vi "SetClipboardData.vi"(4 "error in (no error)":errorcluster, 6 "Format (CF_TEXT)":T1, 7 "hMem":i32 format="%.0x") -> (0 "error out":errorcluster, 3 "hData":i32 format="%.0x")   [LabVIEW 2011]
uses:
  Clipboard Formats.ctl
  KERNEL32.DLL
  user32.dll
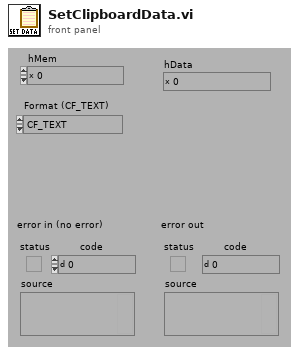
[diagram p1: front panel]
types:
  T1 = typedef "Clipboard Formats.ctl" = enum16{"CF_TEXT"}
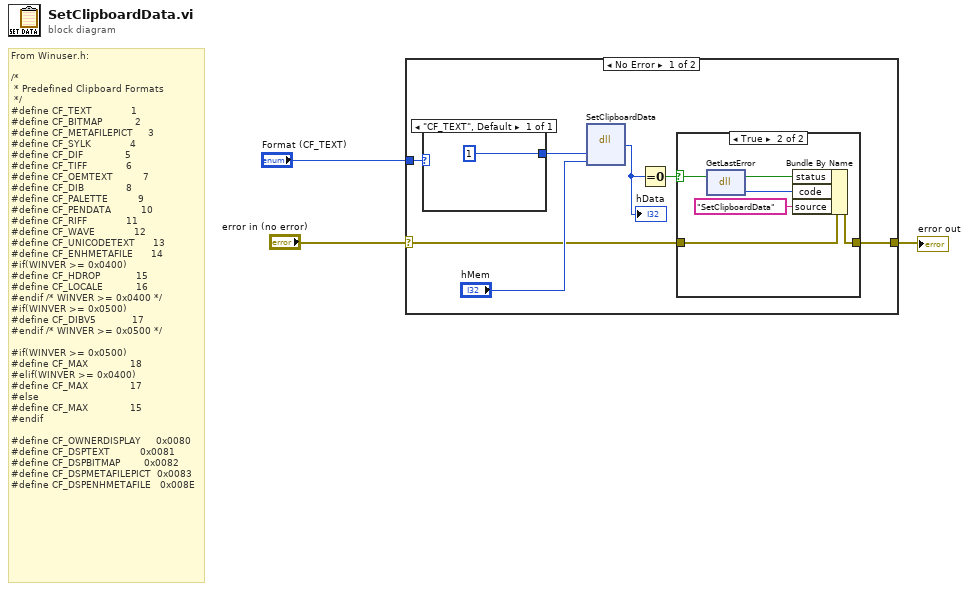
[diagram p0: block diagram]
diagram:
  # "From Winuser.h:\n\n/*\n * Predefined Clipboard Formats\n */\n#define CF_TEXT             1\n#define CF_BITMAP           2\n#define CF_METAFILEPICT     3\n#define CF_SYLK             4\n#define CF_DIF              5\n#define CF_TIFF             6\n#define CF_OEMTEXT          7\n#define CF_DIB              8\n#define CF_PALETTE          9\n#define CF_PENDATA          10\n#define CF_RIFF             11\n#define CF_WAVE             12\n#define CF_UNICODETEXT      13\n#define CF_ENHMETAFILE      14\n#if(WINVER >= 0x0400)\n#define CF_HDROP            15\n#define CF_LOCALE           16\n#endif /* WINVER >= 0x0400 */\n#if(WINVER >= 0x0500)\n#define CF_DIBV5            17\n#endif /* WINVER >= 0x0500 */\n\n#if(WINVER >= 0x0500)\n#define CF_MAX              18\n#elif(WINVER >= 0x0400)\n#define CF_MAX              17\n#else\n#define CF_MAX              15\n#endif\n\n#define CF_OWNERDISPLAY     0x0080\n#define CF_DSPTEXT          0x0081\n#define CF_DSPBITMAP        0x0082\n#define CF_DSPMETAFILEPICT  0x0083\n#define CF_DSPENHMETAFILE   0x008E"
  n1 = case shown="No Error" "error in (no error)" {
    selector: "error in (no error)" -> [w7 w18]
    tunnel: [w6 w18] -> w2
    tunnel: "Format (CF_TEXT)" -> [w4 _]
    frame No Error {
      n2 = case shown="\"CF_TEXT\", Default" w4 {
        tunnel: [u32 1 ("uFormat")] -> w5
        frame "CF_TEXT", Default {
        }
      }
      n3 = dll-call lib="User32.dll" fn="SetClipboardData" label="unsigned long SetClipboardData(\n     unsigned long uFormat, unsigned long hMem);"("uFormat"=w5, "hMem"="hMem") -> ("hData"=w9:i32)  [unwired: 5 in, 2 out]
      "hData" <- w9
      n4 = Equal To 0?(x=w9) -> (x = 0?=w8:bool)
      n5 = case shown="True" w8 {
        selector: w8 -> [_ w16]
        tunnel: w7 -> [w12 w17]
        tunnel: [w12 w14] -> w6
        frame False {
        }
        frame True {
          n6 = dll-call lib="kernel32.dll" fn="GetLastError"() -> (w13:i32)  [unwired: 3 in, 2 out]
          n7 = Bundle By Name(cluster=w17, "status"=w16, "code"=w13, "source"="SetClipboardData") -> (w14:errorcluster)
        }
      }
    }
    frame Error {
    }
  }
  "error out" <- w2
